vi "Set Database Item Metadata.vi"(8 "error in (no error)":errorcluster, 9 "metadata":string, 10 "database item id":u32, 11 "eLab in":refnum<class "PL eLabFTW Client.lvclass">) -> (0 "error out":errorcluster, 3 "eLab out":refnum<class "PL eLabFTW Client.lvclass">)   [LabVIEW 2015, in "PL eLabFTW Client.lvclass"]
doc: "Sets database item metadata."
uses:
  PL eLabFTW Client.lvclass
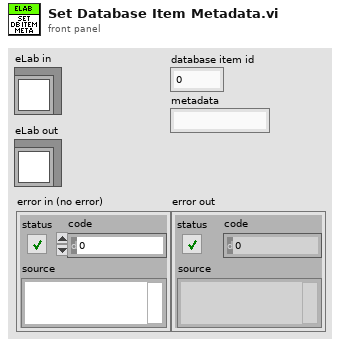
[diagram p1: front panel]
types:
  T1 = cluster{"format string":string, "metadata":string}
  T2 = cluster{"format string":string, "metadata":string}[]
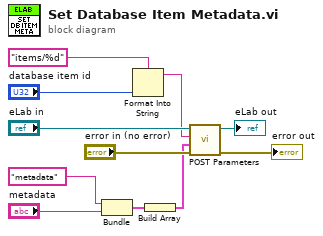
[diagram p0: block diagram]
diagram:
  n1 = Bundle("format string"="metadata", "metadata"="metadata") -> (w4:T1)  [unwired: 1 in]
  n2 = Format Into String(format string="items/%d", "database item id") -> (resulting string=w5:string)  [unwired: 2 in, 1 out]
  n3 = Build Array(w4) -> (w1:T2)
  n4 = call "POST Parameters.vi"("error in (no error)"="error in (no error)", "parameters"=w1, "relative URL"=w5, "eLab in"="eLab in") -> ("error out"=→"error out":errorcluster, "eLab out"=→"eLab out":refnum<class "PL eLabFTW Client.lvclass">)  [unwired: 5 in, 1 out]
